vi "SetChangeSystemSampleTrigger.vi"(0 "controller in":refnum<k24>, 5 "signal":i32(ring)=51 items=["VirtualBinaryInput"=51, "VirtualBinaryOutput"=52, "VirtualRegisterInput"=53, "VirtualRegisterOutput"=54, "Timer"=56, "TimerPerformance"=57, "GlobalVariable"=74, "LibraryCommand"=148, "DataCollectionSampleTime"=149, "DataCollectionSampleIndex"=161, "ZYGOPosition1"=164, "ZYGOPosition2"=165, "ZYGOPosition3"=166, "ZYGOPosition4"=167, "PCModbusMasterConnected"=170, "PCModbusSlaveConnected"=171, "PCModbusMasterErrorCode"=174, "PCModbusSlaveErrorCode"=175, "PCModbusMasterErrorLocation"=176, "PCModbusSlaveErrorLocation"=177, "StopWatchTimer"=197, "ScopetrigID"=209, "PLCBool"=211, "PLCByte"=212, "PLCWord"=213, "PLCDword"=214, "PLCSint"=215, "PLCInt"=216, "PLCDint"=217, "PLCUsint"=218, "PLCUint"=219, "PLCUdint"=220, "PLCReal"=221, "PLCLreal"=222, "EstimatedProcessorUsage"=236, "DataCollectionStatus"=255, "SignalLogState"=270, "FieldbusConnected"=284, "FieldbusErrorCode"=285, "FieldbusErrorLocation"=286, "FieldbusActiveConnections"=287, "FieldbusInactiveConnections"=288, "SafeZoneViolationMask"=289, "SafeZoneActiveMask"=321, "FieldbusInputs"=340, "FieldbusOutputs"=341, "ModbusMasterInputWords"=342, "ModbusMasterOutputWords"=343, "ModbusMasterInputBits"=344, "ModbusMasterOutputBits"=345, "ModbusMasterOutputStatusBits"=346, "ModbusMasterOutputStatusWords"=347, "ModbusSlaveInputWords"=348, "ModbusSlaveOutputWords"=349, "ModbusSlaveInputBits"=350, "ModbusSlaveOutputBits"=351, "DriveModbusMasterInputWords"=352, "DriveModbusMasterOutputWords"=353, "DriveModbusMasterInputBits"=354, "DriveModbusMasterOutputBits"=355, "DriveModbusMasterOutputStatusBits"=356, "DriveModbusMasterOutputStatusWords"=357, "SystemParameter"=379], 9 "optional":i32, 11 "error in (no error)":errorcluster, 12 "trigger":i32(ring)=1 items=["OnAnyChange"=1, "OnIncrease"=2, "OnDecrease"=3]) -> (4 "controller out":refnum<k24>, 15 "error out":errorcluster)   [LabVIEW 2010]
uses:
  c:/aerotech/controller/5.xx.xxx/A3200/pc/labview/2010/bin/Aerotech.A3200.dll
  bin/Aerotech.A3200.dll
  c:/aerotech/controller/5.xx.xxx/A3200/pc/labview/2010/bin/Aerotech.A3200.LabVIEW.dll
  bin/Aerotech.A3200.LabVIEW.dll
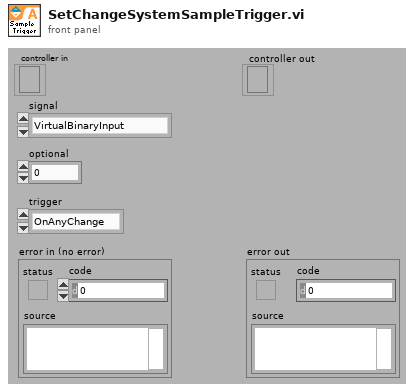
[diagram p1: front panel]
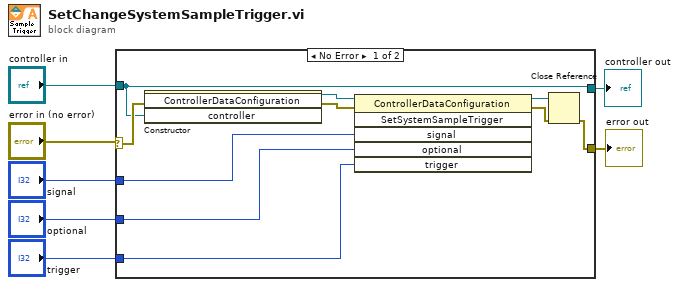
[diagram p0: block diagram]
diagram:
  n1 = case shown="No Error" "error in (no error)" {
    selector: "error in (no error)" -> [w17 w19]
    tunnel: "controller in" -> [w14 w18]
    tunnel: [w11 w19] -> w4
    tunnel: [w14 w18] -> w5
    tunnel: "optional" -> [w10 _]
    tunnel: "trigger" -> [w9 _]
    tunnel: "signal" -> [w8 _]
    frame No Error {
      n2 = constructor class="ControllerDataConfiguration"(error in=w17, "controller"=w14) -> (reference out=w16:refnum<k24>, error out=w15:errorcluster)  [unwired: 2 in, 2 out]
      n3 = invoke class="ControllerDataConfiguration" method="SetSystemSampleTrigger"(reference=w16, error in=w15, "signal"=w8, "optional"=w10, "trigger"=w9) -> (reference out=w12:refnum<k24>, error out=w13:errorcluster)  [unwired: 1 in, 4 out]
      n4 = Close Reference(reference=w12, error in (no error)=w13) -> (error out=w11:errorcluster)
    }
    frame Error {
    }
  }
  "controller out" <- w5
  "error out" <- w4
